vi "Time Estimate.vi"(8 "error in (no error)":errorcluster, 9 "expmode":i32, 10 "scantype":T1(ring), 11 "Wavelength.lvclass":refnum<class "Wavelength Triax 550.lvclass">) -> (0 "error out":errorcluster, 1 "Time Estimate":string, 2 "time":dbl[unit], 3 "Wavelength.lvclass":refnum<class "Wavelength Triax 550.lvclass">)   [LabVIEW 2017, in "Wavelength Triax 550.lvclass"]
uses:
  Wavelength Triax 550.lvclass
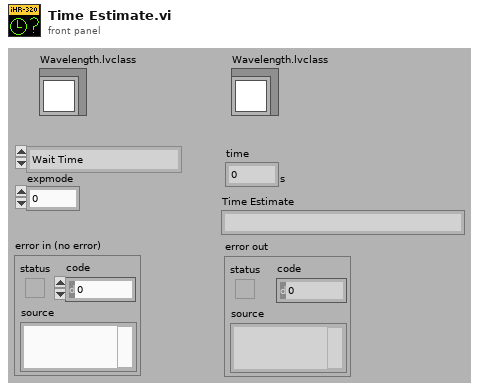
[diagram p1: front panel]
types:
  T1 = enum16{"Wait Time", "Pulse Width", "Wavelength", "Magnetic Field", "rf Scan"}
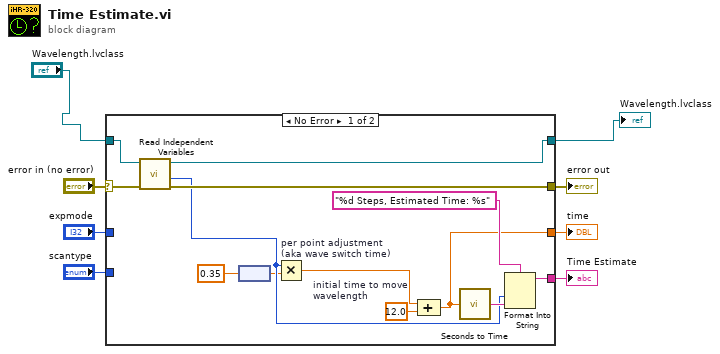
[diagram p0: block diagram]
diagram:
  n1 = case shown="No Error" "error in (no error)" {
    selector: "error in (no error)" -> [w18 w22]
    tunnel: [w13 _] -> w3
    tunnel: "expmode" -> [_ _]
    tunnel: "scantype" -> [_ _]
    tunnel: [w11 _] -> w6
    tunnel: [w19 w23] -> w2
    tunnel: "Wavelength.lvclass" -> [w20 w23]
    tunnel: [w21 w22] -> w5
    frame No Error {
      w17 = dbl[unit] 12.0  # initial time to move wavelength
      n2 = call-dynamic "Read Independent Variables.vi"("error in (no error)"=w18, "Scanner.lvclass in"=w20) -> ("error out"=w21:errorcluster, "size"=w14:i32, "Scanner.lvclass out"=w19:refnum<class "Wavelength Triax 550.lvclass">)  [unwired: 7 out]
      n3 = node(0.35) -> (w9:dbl[unit])
      n4 = Multiply "per point adjustment\n(aka wave switch time)"(x=w14, y=w9) -> (x*y=w12:dbl[unit])
      n5 = Compound Arithmetic op=ADD(w12, w17) -> (w11:dbl[unit])
      n6 = call "Seconds to Time.vi"("Seconds"=w11) -> ("Time"=w15:string)
      n7 = Format Into String(format string="%d Steps, Estimated Time: %s", w14, w15) -> (resulting string=w13:string)  [unwired: 2 in, 1 out]
    }
    frame Error {
    }
  }
  "time" <- w6
  "error out" <- w5
  "Time Estimate" <- w3
  "Wavelength.lvclass" <- w2
